vi "SysDef.Property.Get.Path.vi"(8 "error in (no error)":errorcluster, 9 "Value":path, 10 "Property Name":string, 11 "nodeID":u64) -> (0 "error out":errorcluster, 1 "Value out":path, 3 "nodeID out":u64, 4 "Found?":bool)   [LabVIEW 2027, in "Advanced System Definition.lvlib"]
uses:
  SysDef API/Advanced System Definition.lvlib
  <vilib>/NI VeriStand/Custom Device API/Get Item Property (Path).vi
  C:/NetCore/niveristand-custom-device-development-tools/advanced-sysdef-api/Source/_SubVIs/SysDef.Property.Get.Path.vi/NationalInstruments.VeriStand.SystemDefinitionAPI
  NationalInstruments.VeriStand.SystemDefinitionAPI
  <vilib>/NI VeriStand/Custom Device API/Custom Device API.lvlib
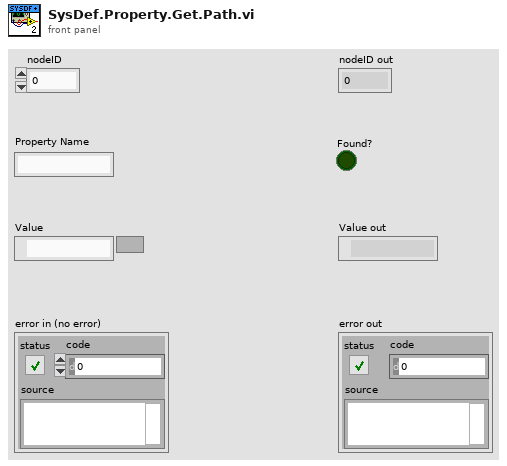
[diagram p1: front panel]
types:
  T1 = typedef "Custom Device API.lvlib/Custom Device Item Ref.ctl" = u64
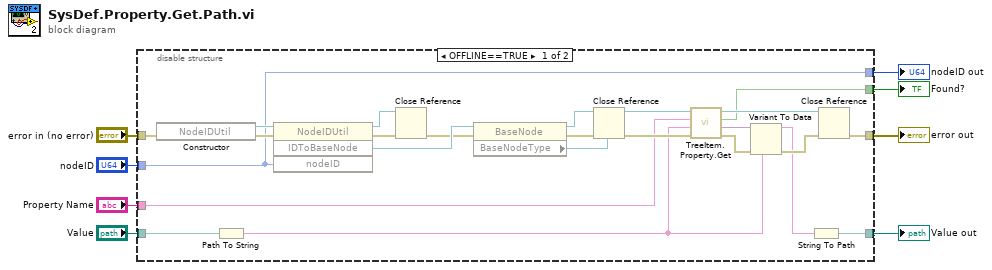
[diagram p0: block diagram]
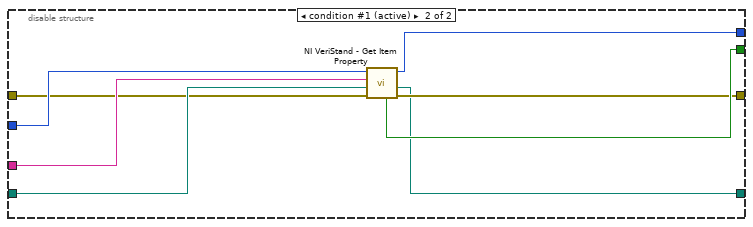
[diagram p2: hidden frame]
diagram:
  n1 = disable-structure shown="OFFLINE==TRUE" {
    disable-tunnel: "error in (no error)" -> [w24 w36]
    disable-tunnel: "nodeID" -> [w13 w37]
    disable-tunnel: [w19 w34] -> w6
    disable-tunnel: "Property Name" -> [w18 w38]
    disable-tunnel: [w14 w35] -> w4
    disable-tunnel: "Value" -> [w12 w39]
    disable-tunnel: [w9 w32] -> w2
    disable-tunnel: [w13 w33] -> w1
    frame condition #0 {
      n2 = constructor class="NodeIDUtil"(error in=w24) -> (reference out=w31:refnum<k24>, error out=w30:errorcluster)  [unwired: 2 in, 1 out]
      n3 = Path To String(path=w12) -> (string=w11:string)
      n4 = invoke class="NodeIDUtil" method="IDToBaseNode"(reference=w31, error in=w30, "nodeID"=w13) -> (reference out=w25:refnum<k24>, error out=w27:errorcluster, "IDToBaseNode"=w29:refnum<k24>)  [unwired: 1 in, 1 out]
      n5 = Close Reference(reference=w25, error in (no error)=w27) -> (error out=w26:errorcluster)
      n6 = property class="BaseNode"(reference=w29, error in=w26) -> (reference out=w23:refnum<k24>, error out=w22:errorcluster, "BaseNodeType"=w28:refnum<k24>)
      n7 = Close Reference(reference=w23, error in (no error)=w22) -> (error out=w21:errorcluster)
      n8 = call "TreeItem.Property.Get.vi"("error in (no error)"=w21, "Default Value"=w11, "Property Name"=w18, "NationalInstruments.VeriStand.SystemStorage.BaseNodeType"=w28) -> ("error out"=w16:errorcluster, "Variant"=w17:variant, "Found?"=w14:bool, "NationalInstruments.VeriStand.SystemStorage.BaseNodeType"=w20:refnum<k39>)  [unwired: 4 in]
      n9 = Variant To Data(error in=w16, type=w11, Variant=w17) -> (data=w10:string, error out=w15:errorcluster)
      n10 = String To Path(string=w10) -> (path=w9:path)
      n11 = Close Reference(reference=w20, error in (no error)=w15) -> (error out=w19:errorcluster)
    }
    frame condition #1 (active) {
      n12 = call-poly <vilib>:"NI VeriStand - Get Item Property.vi"("error in (no error)"=w36, "Default Value"=w39, "Property Name"=w38, "Item Ref in"=w37) -> ("error out"=w34:errorcluster, "Value"=w32:path, "Item Ref out"=w33:T1, "Found?"=w35:bool)  [unwired: 4 in]
    }
  }
  "nodeID out" <- w1
  "error out" <- w6
  "Value out" <- w2
  "Found?" <- w4
